vi "User Interface.vi"() -> ()   [LabVIEW 2013]
panel:
  in  "Fan on?":bool
  out "Lamp Intensity":dbl(slide) scale=0.0..100.0
  out "Temperature":dbl(graph)
  in  "Setpoint":dbl(slide)=25.0 scale=20.0..40.0
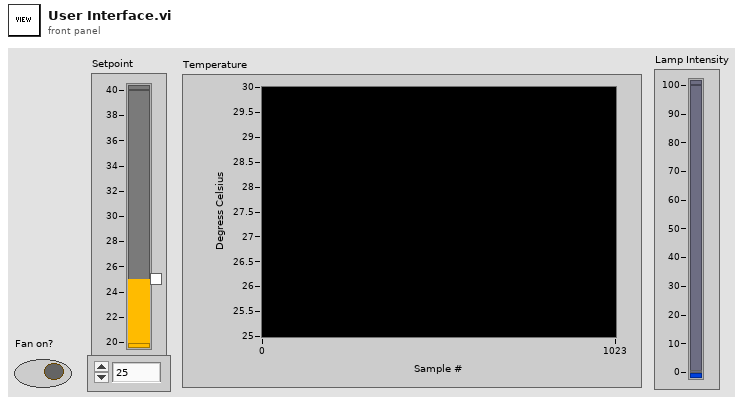
[diagram p1: front panel]
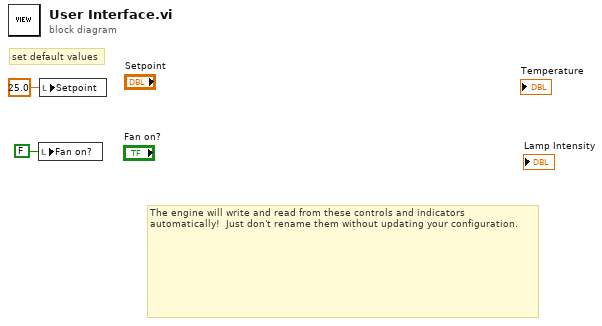
[diagram p0: block diagram]
diagram:
  # "set default values"
  # "The engine will write and read from these controls and indicators automatically!  Just don't rename them without updating your configuration."
  n1 = local write "Fan on?"(FALSE ("Fan on?")) -> ()
  n2 = local write "Setpoint"(25.0 ("Setpoint")) -> ()
